vi "IHL_Update Loop Data.vi"(8 "error in (no error)":errorcluster, 10 "Inspect Helper Loop Data":T1={"IHL State"=enum."Init", "Timeout"=0, "Loop Count"=0, "Start Sample No."=0, "Collecting Data"=FALSE, "No. Samples"=0, "Success Flag"=FALSE, "Inspect Status "={"Ready"=FALSE, "Inspecting"=FALSE, "Cancel"=FALSE}, "Status"=0, "Encoder Count"=0, "PosToStartScan"=50800, "ScanLength"=50800, "MaxSamples"=50800, "PosToEndScan"=0, "Host SampleData"=refnum, "data value reference"=refnum, "Block Cnt notifier out"=refnum, "EventLog"=refnum}, 11 "Tool Status notifier":refnum<notifier>) -> (0 "error out":errorcluster, 2 "Inspect Helper Loop Data out":T1={"IHL State"=enum."Init", "Timeout"=0, "Loop Count"=0, "Start Sample No."=0, "Collecting Data"=FALSE, "No. Samples"=0, "Success Flag"=FALSE, "Inspect Status "={"Ready"=FALSE, "Inspecting"=FALSE, "Cancel"=FALSE}, "Status"=0, "Encoder Count"=0, "PosToStartScan"=50800, "ScanLength"=50800, "MaxSamples"=50800, "PosToEndScan"=0, "Host SampleData"=refnum, "data value reference"=refnum, "Block Cnt notifier out"=refnum, "EventLog"=refnum})   [LabVIEW 2015, in "Tool Module.lvlib"]
uses:
  Tool Module.lvlib
  _IHL Status Notifier Data Cluster--typedef.ctl
  _IHL Data Cluster--typedef.ctl
  Event Logger Library/Event Log/EventLog.lvclass
  _IHL SM Enum--typedef.ctl
  _IHL Status Update Cluster--typedef.ctl
  _Sample Data Rtn Cluster--typedef.ctl
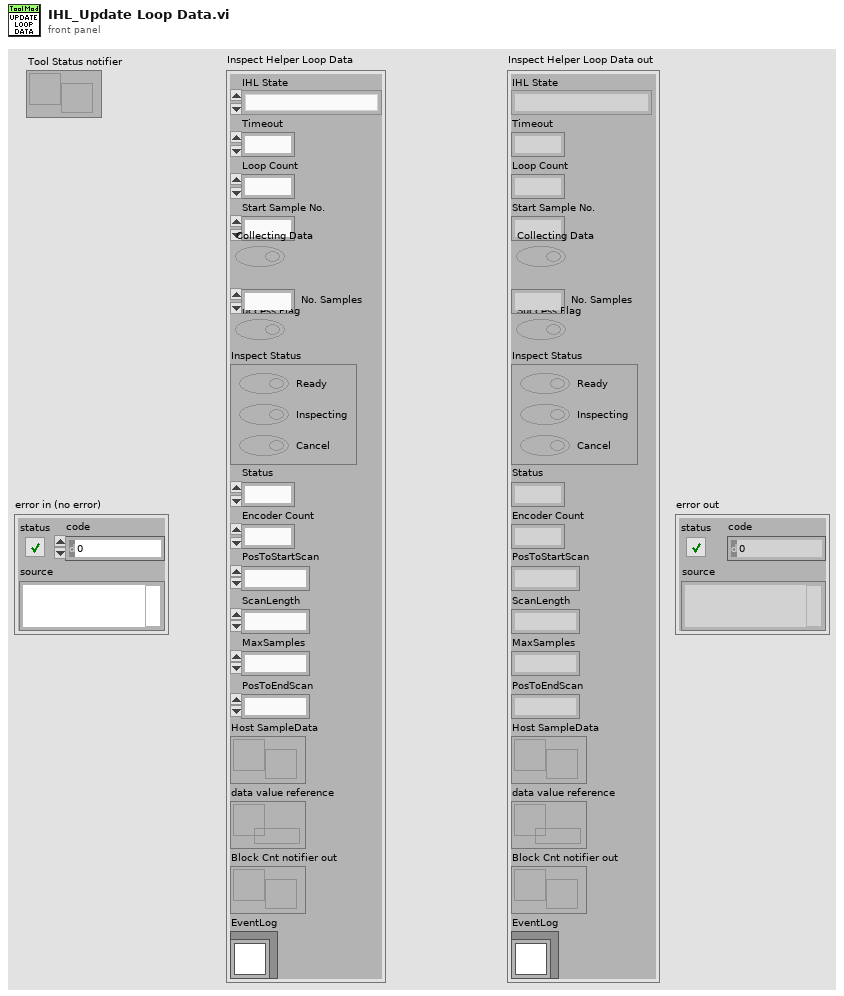
[diagram p1: front panel]
types:
  T1 = typedef "Tool Module.lvlib/_IHL Data Cluster--typedef.ctl" = cluster{"IHL State":T2, "Timeout":i32, "Loop Count":i32, "Start Sample No.":u32, "Collecting Data":bool, "No. Samples":i32, "Success Flag":bool, "Inspect Status ":T3, "Status":u16, "Encoder Count":i32, "PosToStartScan":i32, "ScanLength":i32, "MaxSamples":i32, "PosToEndScan":i32, "Host SampleData":refnum<notifier>, "data value reference":refnum<data-value>, "Block Cnt notifier out":refnum<notifier>, "EventLog":refnum<class "EventLog.lvclass">}
  T2 = typedef "Tool Module.lvlib/_IHL SM Enum--typedef.ctl" = enum16{"Init", "Set Motion Speed", "Move To Scan Start", "Wait for Motion Out", "Wait for Start Pos", "Inspect: START", "Wait for Motion IN", "Wait for Inspect Range", "Inspecting", "Inspect: STOP"}
  T3 = typedef "Tool Module.lvlib/_IHL Status Update Cluster--typedef.ctl" = cluster{"Ready":bool, "Inspecting":bool, "Cancel":bool}
  T4 = typedef "Tool Module.lvlib/_IHL Status Notifier Data Cluster--typedef.ctl" = cluster{"Status":u16, "Encoder":i32}
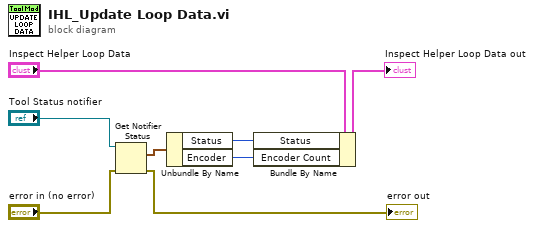
[diagram p0: block diagram]
diagram:
  n1 = Get Notifier Status(notifier="Tool Status notifier", error in (no error)="error in (no error)") -> (current notification=w4:T4, error out=→"error out":errorcluster)  [unwired: 3 out]
  n2 = Unbundle By Name(w4) -> ("Status"=w3:u16, "Encoder"=w2:i32)
  n3 = Bundle By Name(cluster="Inspect Helper Loop Data", "Status"=w3, "Encoder Count"=w2) -> (→"Inspect Helper Loop Data out":T1)
